vi "Path to Icons Folder.vi"(8 "Error In":errorcluster) -> (0 "Error Out":errorcluster, 3 "Path to Icons Folder":path)   [LabVIEW 2014]
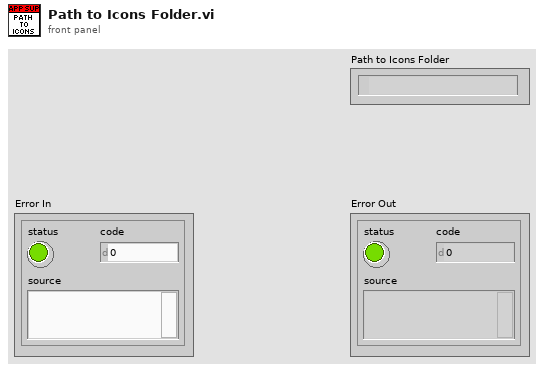
[diagram p1: front panel]
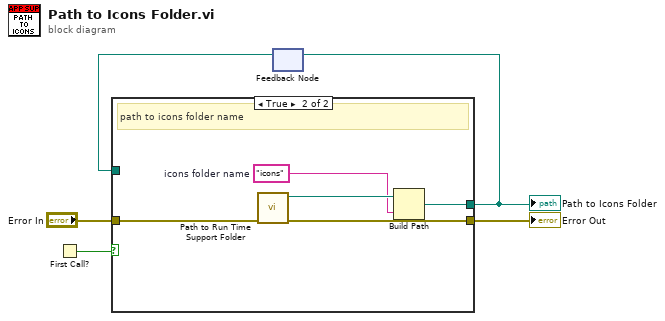
[diagram p0: block diagram]
diagram:
  n1 = First Call?() -> (First Call?: T/F=w1:bool)
  n2 = feedback #1() -> (w2:path)  [unwired: 1 in]
  n3 = case shown="True" w1 {
    tunnel: "Error In" -> [w6 w11]
    tunnel: [w6 w9] -> w4
    tunnel: [w7 w8] -> w3
    tunnel: w2 -> [w7 _]
    frame False {
      # "return path"
    }
    frame True {
      w10 = "icons"  # icons folder name
      # "path to icons folder name"
      n4 = call "Path to Run Time Support Folder.vi"("Error In"=w11) -> ("Error Out"=w9:errorcluster, "Path To Run Time Support Folder"=w12:path)  [unwired: 9 in]
      n5 = Build Path(base path=w12, name or relative path=w10) -> (appended path=w8:path)
    }
  }
  "Error Out" <- w4
  "Path to Icons Folder" <- w3
  n6 = feedback-in #1(w3) -> ()
